vi "Write_parameter.vi"(8 "error in (no error)":errorcluster caption="entrée d'erreur (pas d'erreur)", 10 "Parameter":string, 11 "Class Instrument Multimeter en entrée":refnum<class "Class Instrument Balance.lvclass">) -> (0 "error out":errorcluster caption="sortie d'erreur", 3 "Class Instrument Multimeter en sortie":refnum<class "Class Instrument Balance.lvclass">)   [LabVIEW 2020, in "Library Instrument & Equipement.lvlib" / "Library Instruments.lvlib" / "Class Instrument Balance.lvclass"]
uses:
  Class Instrument Balance.lvclass
  Commun VI/TypeDef/Commande Balance/Parameter Balance.ctl
  Balance/Balance (Default)/Class Balance (Default).lvclass
  JSON API/JSON Value/Set from JSON string.vi
  Instrument (Default)/Class Instrument (Default).lvclass
  JSON API/JSON Value/JSON Value.lvclass
  Class Instrument Balance.lvclass/Class Instrument Balance.ctl
  JSON API/Variant JSON/Variant JSON.lvlib
  JSON API/Get Polymorphic/JSON GetSet.lvlib
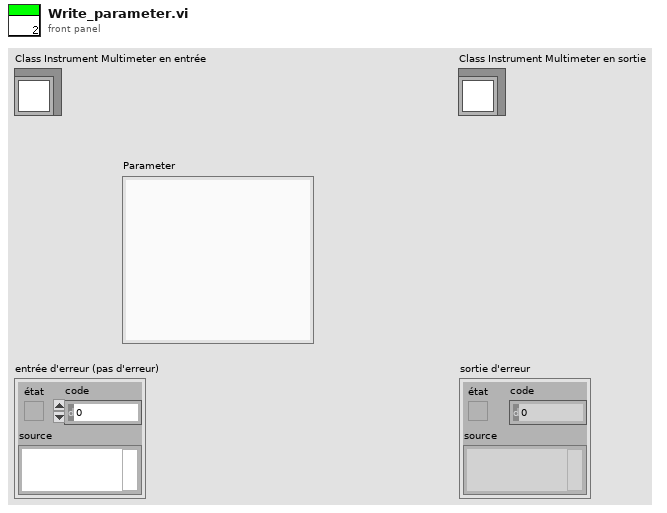
[diagram p1: front panel]
types:
  T1 = typedef "Parameter Balance.ctl" = cluster{"Device @":string, "Timeout":u32, "Class Balance":refnum<class "Class Balance (Default).lvclass">}
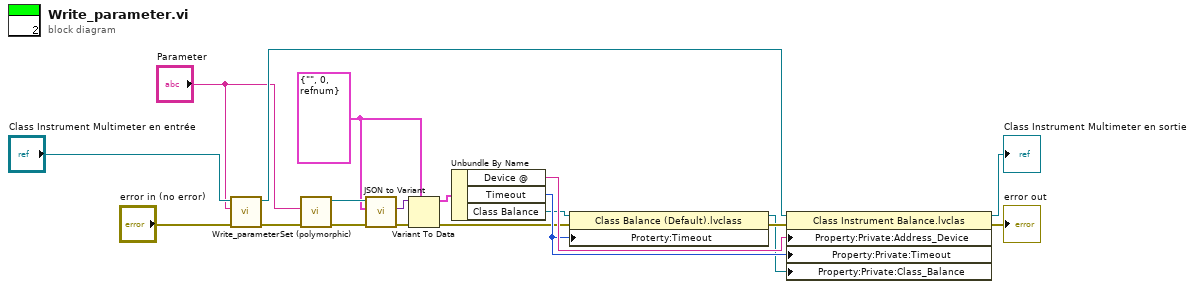
[diagram p0: block diagram]
diagram:
  w6 = T1 {"Device @"="", "Timeout"=0, "Class Balance"=refnum} ("Parameter")
  n1 = call-parent "Write_parameter.vi"("error in (no error)"="error in (no error)", "Parameter"="Parameter", "Class Instrument (Default) en entrée"="Class Instrument Multimeter en entrée") -> ("error out"=w10:errorcluster, "Class Instrument (Default) en sortie"=w9:refnum<class "Class Instrument Balance.lvclass">)  [unwired: 7 in]
  n2 = call-poly "Set (polymorphic).vi"("error in (no error)"=w10, "JSON stream"="Parameter") -> ("error out"=w17:errorcluster, "JSON Value out"=w19:refnum<class "JSON Value.lvclass">)  [unwired: 7 in, 1 out]
  n3 = call "JSON to Variant.vi"("error in (no error)"=w17, "Variant (Data Type)"=w6, "JSON Value"=w19) -> ("error out"=w18:errorcluster, "Variant out"=w16:variant)  [unwired: 7 in]
  n4 = Variant To Data(error in=w18, type=w6, Variant=w16) -> (data=w13:T1, error out=w3:errorcluster)
  n5 = Unbundle By Name(w13) -> ("Device @"=w12:string, "Timeout"=w5:u32, "Class Balance"=w4:refnum<class "Class Balance (Default).lvclass">)
  n6 = property class="Class Balance (Default).lvclass"(reference=w4, error in=w3, "Proterty:Timeout"=w5) -> (reference out=w1:refnum<class "Class Balance (Default).lvclass">, error out=w2:errorcluster)
  n7 = property class="Class Instrument Balance.lvclas"(reference=w9, error in=w2, "Property:Private:Address_Device"=w12, "Property:Private:Timeout"=w5, "Property:Private:Class_Balance"=w1) -> (reference out=→"Class Instrument Multimeter en sortie":refnum<class "Class Instrument Balance.lvclass">, error out=→"error out":errorcluster)
